vi "Initialize Front Panel.vi"(8 "error in (no error)":errorcluster, 11 "Login View in":refnum<class "Login View.lvclass">) -> (0 "error out":errorcluster, 3 "Login View out":refnum<class "Login View.lvclass">)   [LabVIEW 2017, in "Login View.lvlib" / "Login View.lvclass"]
doc: "<License>\nCopyright © 2017 Composed Systems, LLC | All rights reserved\nwww.composed.io\n\nAuthor: Ethan Stern <ethan.stern@composed.io>\n\nThis software is provided \"AS IS\" WITHOUT WARRANTIES, either express or implied, AND IS FOR EDUCATIONAL PURPOSES ONLY.\n</License>"
uses:
  Login View.lvclass
  Login View.lvclass/Login View.ctl
  User Manager Model/Type Definitions/Credentials.ctl
  <vilib>/gpm_packages/@cs/mva-viewable/Source/IViewable/IViewable/IViewable.lvclass
  User Manager Model/Type Definitions/User Manager Application Types.lvlib
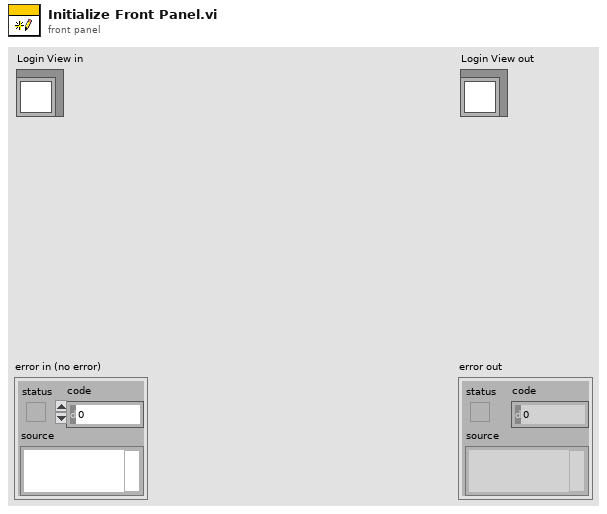
[diagram p1: front panel]
types:
  T1 = enum8{"Enabled", "Disabled", "Disabled and Grayed Out"}
  T2 = typedef "User Manager Application Types.lvlib/Credentials.ctl" = cluster{"Username":string, "Password":string}
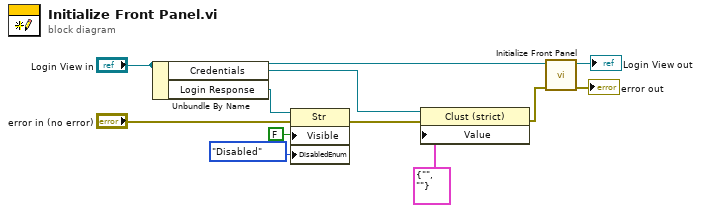
[diagram p0: block diagram]
diagram:
  n1 = Unbundle By Name("Login View in") -> ("Credentials"=w5:refnum<vi>, "Login Response"=w8:refnum<vi>)
  n2 = property class="Str"(reference=w8, error in="error in (no error)", "Visible"=FALSE, "DisabledEnum"=T1."Disabled" ("Disabled")) -> (error out=w3:errorcluster)  [unwired: 1 out]
  n3 = property class="Clust (strict)"(reference=w5, error in=w3, "Value"=T2 {"Username"="", "Password"=""}) -> (error out=w2:errorcluster)  [unwired: 1 out]
  n4 = call-parent "Initialize Front Panel.vi"("error in (no error)"=w2, "IViewable in"="Login View in") -> ("error out"=→"error out":errorcluster, "IViewable out"=→"Login View out":refnum<class "Login View.lvclass">)  [unwired: 8 in]
